vi "Configure Detection Mode.vi"(0 "VISA resource name":refnum<visa-resource-name>, 5 "Detection Mode (0:Normal)":i32(ring) items=["Normal", "Positive", "Sample", "Negative", "RMS", "QP", "CISPR", "CRMS"], 11 "error in (no error)":errorcluster) -> (4 "VISA resource name out":refnum<visa-resource-name>, 15 "error out":errorcluster)   [LabVIEW 2020, in "Anritsu Signal Analyzer Series.lvlib"]
doc: "Configures the Detection Mode settings of the spectrum analyzer."
uses:
  Anritsu Signal Analyzer Series.lvlib
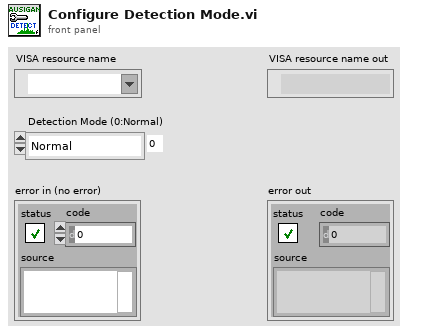
[diagram p1: front panel]
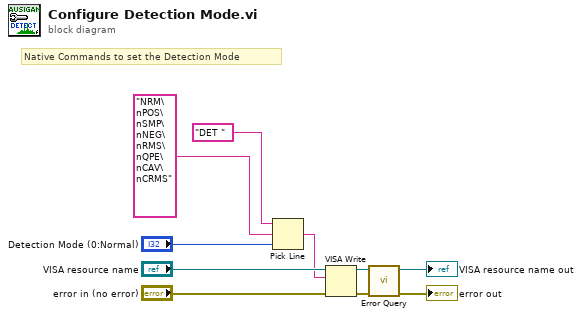
[diagram p0: block diagram]
diagram:
  # "Native Commands to set the Detection Mode"
  n1 = Pick Line(string ("")="DET " ("_Command Set"), multi-line string="NRM\nPOS\nSMP\nNEG\nRMS\nQPE\nCAV\nCRMS" ("複数行文字列"), line index="Detection Mode (0:Normal)") -> (output string=w1:string)
  n2 = VISA Write(VISA resource name="VISA resource name", write buffer=w1, error in (no error)="error in (no error)") -> (VISA resource name out=w4:refnum<visa-resource-name>, error out=w5:errorcluster)  [unwired: 1 out]
  n3 = call "Error Query.vi"("error in (no error)"=w5, "VISA resource name"=w4) -> ("error out"=→"error out":errorcluster, "VISA resource name out"=→"VISA resource name out":refnum<visa-resource-name>)  [unwired: 6 in, 2 out]
